vi "PPS Configure.vi"(8 "error in":errorcluster, 10 "Configure":T1={"Voltage Level (0.0 V)"=0.0, "CURRent Limit (0.0 A)"=0.0, "OVP LEVEL (0V)"=0.0, "OCP LEVEL (0A)"=0.0, "Enable OVP (T: Enable)"=TRUE, "Enable OCP (T: Enable)"=TRUE, "Enable Output "=TRUE, "Delays OCP"=0.0, "Delays OVP"=0.0, "Mode(0:Voltage)"=0, "CURRent Level (0.0 A)"=0.0, "Voltage Limit (0.0 V)"=0.0} {"Voltage Limit (0.0 V)" format="%.2f"; "Mode(0:Voltage)" items=["Voltage", "Current"]; "OCP LEVEL (0A)" format="%.2f"; "OVP LEVEL (0V)" format="%.2f"; "Voltage Level (0.0 V)" format="%.2f"}, 11 "IT-M6018C in":refnum<class "IT-M6018C.lvclass">) -> (0 "error out":errorcluster, 3 "IT-M6018C out":refnum<class "IT-M6018C.lvclass">)   [LabVIEW 2023, in "HardwareAbstractionLayer_LVOOP.lvlib" / "IT-M6018C.lvclass"]
uses:
  IT-M6018C.lvclass
  Control/PPS Configure Data.ctl
  <instrlib>/IT6000C/IT6000C.lvlib
  PowerSupply.lvclass
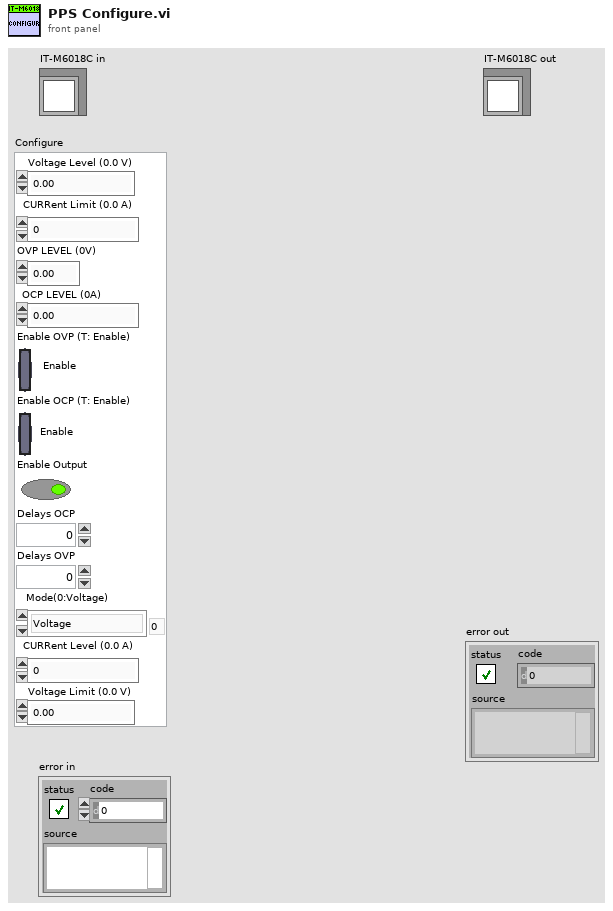
[diagram p1: front panel]
types:
  T1 = typedef "HardwareAbstractionLayer_LVOOP.lvlib/PowerSupply.lvclass/PPS Configure Data.ctl" = cluster{"Voltage Level (0.0 V)":dbl, "CURRent Limit (0.0 A)":dbl, "OVP LEVEL (0V)":dbl, "OCP LEVEL (0A)":dbl, "Enable OVP (T: Enable)":bool, "Enable OCP (T: Enable)":bool, "Enable Output ":bool, "Delays OCP":dbl, "Delays OVP":dbl, "Mode(0:Voltage)":u16, "CURRent Level (0.0 A)":dbl, "Voltage Limit (0.0 V)":dbl}
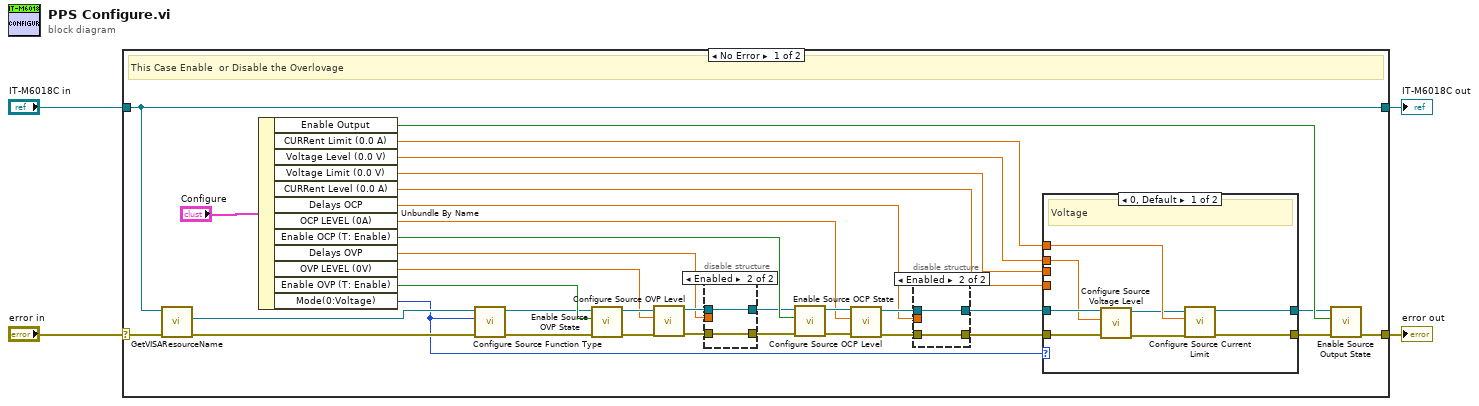
[diagram p0: block diagram]
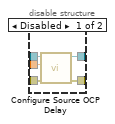
[diagram p2: hidden frame]
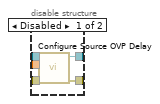
[diagram p3: hidden frame]
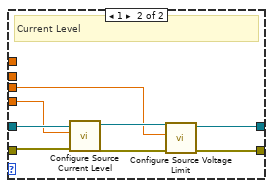
[diagram p4: hidden frame]
diagram:
  n1 = case shown="No Error" "error in" {
    selector: "error in" -> [w26 w69]
    tunnel: [w34 w69] -> w3
    tunnel: "IT-M6018C in" -> [w25 w70]
    tunnel: [w25 w70] -> w1
    frame No Error {
      # "This Case Enable  or Disable the Overlovage"
      n2 = call "GetVISAResourceName.vi"("error in (no error)"=w26, "object in"=w25) -> ("error out"=w22:errorcluster, "VISA resource name"=w24:refnum<visa-resource-name>)  [unwired: 7 in, 1 out]
      n3 = Unbundle By Name("Configure") -> ("Enable Output"=w27:bool, "CURRent Limit (0.0 A)"=w18:dbl, "Voltage Level (0.0 V)"=w28:dbl, "Voltage Limit (0.0 V)"=w15:dbl, "CURRent Level (0.0 A)"=w19:dbl, "Delays OCP"=w5:dbl, "OCP LEVEL (0A)"=w29:dbl, "Enable OCP (T: Enable)"=w30:bool, "Delays OVP"=w10:dbl, "OVP LEVEL (0V)"=w31:dbl, "Enable OVP (T: Enable)"=w32:bool, "Mode(0:Voltage)"=w20:u16)
      n4 = call <instrlib>:"Configure Source Function Type.vi"("error in (no error)"=w22, "Mode(0:Voltage)"=w20, "VISA resource name"=w24) -> ("error out"=w21:errorcluster, "VISA resource name out"=w23:refnum<visa-resource-name>)  [unwired: 7 in]
      n5 = call <instrlib>:"Enable Source OVP State.vi"("error in (no error)"=w21, "Enable(True)"=w32, "VISA resource name"=w23) -> ("error out"=w38:errorcluster, "VISA resource name out"=w37:refnum<visa-resource-name>)  [unwired: 7 in]
      n6 = call <instrlib>:"Configure Source OVP Level.vi"("error in (no error)"=w38, "Value(0)"=w31, "VISA resource name"=w37) -> ("error out"=w12:errorcluster, "VISA resource name out"=w14:refnum<visa-resource-name>)  [unwired: 7 in]
      n7 = disable-structure shown="Enabled" {
        disable-tunnel: w14 -> [w50 w52]
        disable-tunnel: [w49 w52] -> w13
        disable-tunnel: w12 -> [w48 w51]
        disable-tunnel: [w47 w51] -> w11
        disable-tunnel: w10 -> [w46 _]
        frame Disabled {
          n8 = call <instrlib>:"Configure Source OVP Delay.vi"("error in (no error)"=w48, "Value(0)"=w46, "VISA resource name"=w50) -> ("error out"=w47:errorcluster, "VISA resource name out"=w49:refnum<visa-resource-name>)  [unwired: 7 in]
        }
        frame Enabled {
        }
      }
      n9 = call <instrlib>:"Enable Source OCP State.vi"("error in (no error)"=w11, "Enable(True)"=w30, "VISA resource name"=w13) -> ("error out"=w35:errorcluster, "VISA resource name out"=w36:refnum<visa-resource-name>)  [unwired: 7 in]
      n10 = call <instrlib>:"Configure Source OCP Level.vi"("error in (no error)"=w35, "Value(0)"=w29, "VISA resource name"=w36) -> ("error out"=w9:errorcluster, "VISA resource name out"=w7:refnum<visa-resource-name>)  [unwired: 7 in]
      n11 = disable-structure shown="Enabled" {
        disable-tunnel: w9 -> [w43 w44]
        disable-tunnel: [w42 w44] -> w8
        disable-tunnel: w7 -> [w41 w45]
        disable-tunnel: [w40 w45] -> w6
        disable-tunnel: w5 -> [w39 _]
        frame Disabled {
          n12 = call <instrlib>:"Configure Source OCP Delay.vi"("error in (no error)"=w43, "Value(0)"=w39, "VISA resource name"=w41) -> ("error out"=w42:errorcluster, "VISA resource name out"=w40:refnum<visa-resource-name>)  [unwired: 7 in]
        }
        frame Enabled {
        }
      }
      n13 = case shown="0, Default" w20 {
        tunnel: w6 -> [w60 w68]
        tunnel: w8 -> [w59 w67]
        tunnel: w28 -> [w58 _]
        tunnel: w19 -> [_ w66]
        tunnel: w18 -> [w56 _]
        tunnel: [w54 w63] -> w17
        tunnel: [w53 w62] -> w16
        tunnel: w15 -> [_ w61]
        frame 0, Default {
          # "Voltage"
          n14 = call <instrlib>:"Configure Source Voltage Level.vi"("error in (no error)"=w59, "Value(0)"=w58, "VISA resource name"=w60) -> ("error out"=w57:errorcluster, "VISA resource name out"=w55:refnum<visa-resource-name>)  [unwired: 7 in]
          n15 = call <instrlib>:"Configure Source Current Limit.vi"("error in (no error)"=w57, "Value(0)"=w56, "VISA resource name"=w55) -> ("error out"=w54:errorcluster, "VISA resource name out"=w53:refnum<visa-resource-name>)  [unwired: 7 in]
        }
        frame 1 {
          # "Current Level"
          n16 = call <instrlib>:"Configure Source Current Level.vi"("error in (no error)"=w67, "Value(0)"=w66, "VISA resource name"=w68) -> ("error out"=w64:errorcluster, "VISA resource name out"=w65:refnum<visa-resource-name>)  [unwired: 7 in]
          n17 = call <instrlib>:"Configure Source Voltage Limit.vi"("error in (no error)"=w64, "Value(0)"=w61, "VISA resource name"=w65) -> ("error out"=w63:errorcluster, "VISA resource name out"=w62:refnum<visa-resource-name>)  [unwired: 7 in]
        }
      }
      n18 = call <instrlib>:"Enable Source Output State.vi"("error in (no error)"=w17, "Enable(True)"=w27, "VISA resource name"=w16) -> ("error out"=w34:errorcluster)  [unwired: 7 in, 1 out]
    }
    frame Error {
    }
  }
  "error out" <- w3
  "IT-M6018C out" <- w1
